vi "当前结果保存.vi"(9 "列表2":refnum<vi>, 10 "列表1":refnum<vi>, 11 "保存计数":u32) -> ()   [LabVIEW 2020]
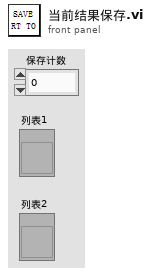
[diagram p1: front panel]
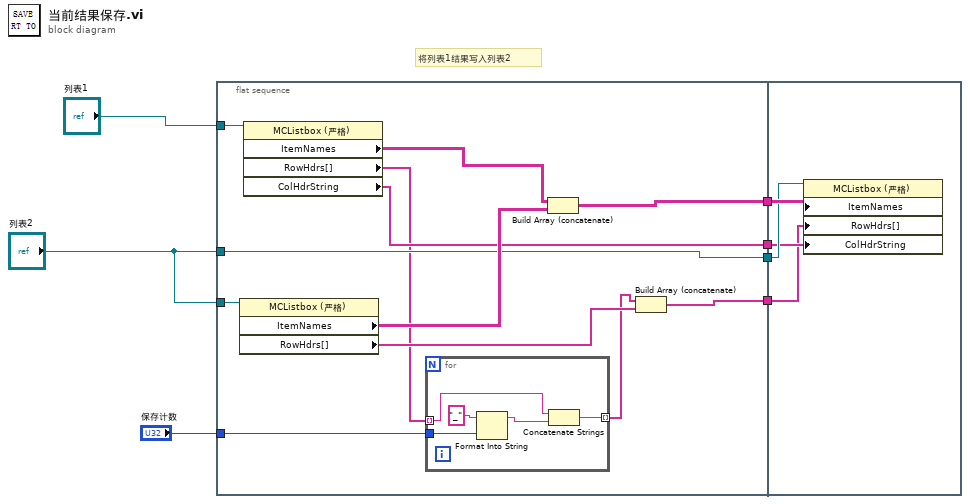
[diagram p0: block diagram]
diagram:
  # "将列表1结果写入列表2"
  n1 = flat-sequence {
    tunnel: "列表1" -> [w17]
    tunnel: "列表2" -> [w16]
    tunnel: [w18] -> w6
    tunnel: [w15] -> w5
    tunnel: "列表2" -> [w15]
    tunnel: [w14] -> w3
    tunnel: [w13] -> w2
    tunnel: "保存计数" -> [w9]
    tunnel: w6 -> [w28]
    tunnel: w5 -> [w27]
    tunnel: w3 -> [w26]
    tunnel: w2 -> [w25]
    frame #0 {
      n2 = property class="MCListbox (严格)"(reference=w16) -> ("ItemNames"=w19:string[][], "RowHdrs[]"=w12:string[])  [unwired: 1 in, 2 out]
      n3 = property class="MCListbox (严格)"(reference=w17) -> ("ItemNames"=w11:string[][], "RowHdrs[]"=w10:string[], "ColHdrString"=w14:string[])  [unwired: 1 in, 2 out]
      n4 = for {
        tunnel: w10 -> [w20] mode=indexing
        tunnel: w9 -> [w24]
        tunnel: [w22] -> w8 mode=indexing
        n5 = Format Into String(initial string="_" ("初始字符串"), w24) -> (resulting string=w21:string)  [unwired: 2 in, 1 out]
        n6 = Concatenate Strings(w20, w21) -> (w22:string)
      }
      n7 = Build Array (concatenate)(w11, w19) -> (w18:string[][])
      n8 = Build Array (concatenate)(w8, w12) -> (w13:string[])
    }
    frame #1 {
      n9 = property class="MCListbox (严格)"(reference=w27, "ItemNames"=w28, "RowHdrs[]"=w25, "ColHdrString"=w26) -> ()  [unwired: 1 in, 2 out]
    }
  }
